vi "Agilent SNA Calibrate.vi"(7 "Agilent SNA & SWP":T6, 8 "error in (no error)":errorcluster, 10 "Parameters to Measure":T2[](array[typedef]) {"Channel" min=1 max=99 step=1; "Parameter"."Stimulus Port" min=1 step=1; "Parameter"."Response Port" min=1 step=1}, 11 "VISA Resource Names":T1) -> (0 "error out":errorcluster {"code" format="%.0x"}, 3 "dup VISA Resource Names":T1)   [LabVIEW 2011]
uses:
  TypeDefs/Agilent SNA VISA.ctl
  TypeDefs/Agilent SNA Instrument Info.ctl
  tests/S Parameter/TypeDefs/SP Parameter to Measure.ctl
  tests/S Parameter/TypeDefs/SP Parameter.ctl
  tests/S Parameter/TypeDefs/SP Calibration State.ctl
  tests/S Parameter/TypeDefs/SP Measurement Format.ctl
  TypeDefs/Agilent SNA Message Mode.ctl
  TypeDefs/Agilent SNA Display Data.ctl
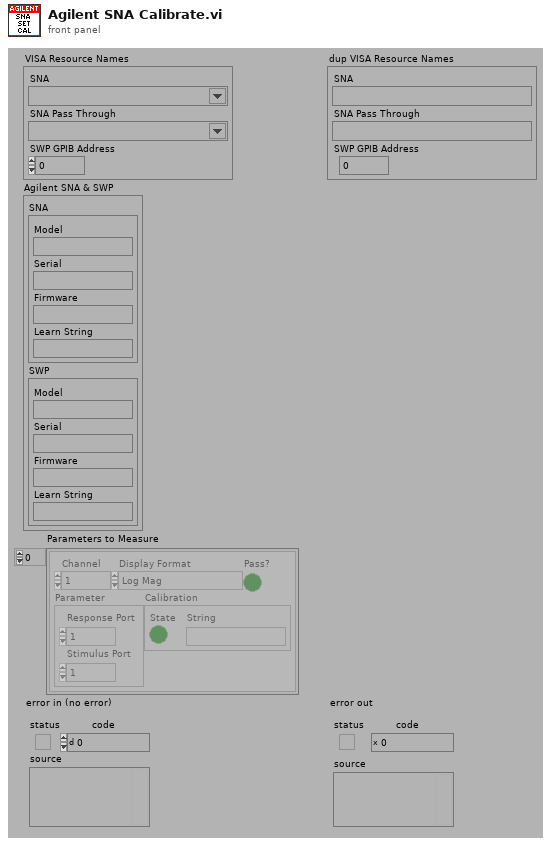
[diagram p1: front panel]
types:
  T1 = typedef "Agilent SNA VISA.ctl" = cluster{"SNA":refnum<visa-resource-name>, "SNA Pass Through":refnum<visa-resource-name>, "SWP GPIB Address":i32}
  T2 = typedef "SP Parameter to Measure.ctl" = cluster{"Channel":i8, "Parameter":T3, "Calibration":T4, "Display Format":T5, "Pass?":bool}
  T3 = typedef "SP Parameter.ctl" = cluster{"Stimulus Port":i8, "Response Port":i8}
  T4 = typedef "SP Calibration State.ctl" = cluster{"State":bool, "String":string}
  T5 = typedef "SP Measurement Format.ctl" = enum32{"Log Mag", "Phase", "Delay", "Smith (R+jX)", "Polar (Re/Im)", "Linear Mag", "SWR", "Real", "Imaginary", "Smith (Lin/Phase)", "Smith (Log/Phase)", "Smith (Real/Imag)", "Smith (G+jB)", "Polar (Lin/Phase)", "Polar (Log/Phase)", "Expanded Phase", "Positive Phase", "Inverted Smith", "Unwrapped Phase", "Power Out", "Power In", "Linear Mag/Phase", "Log Mag/Phase", "Real/Imaginary"}
  T6 = typedef "Agilent SNA Instrument Info.ctl" = cluster{"SNA":cluster{"Model":string, "Serial":string, "Firmware":string, "Learn String":string}, "SWP":cluster{"Model":string, "Serial":string, "Firmware":string, "Learn String":string}}
  T7 = typedef "Agilent SNA Message Mode.ctl" = enum16{"On", "Off"}
  T8 = typedef "Agilent SNA Display Data.ctl" = enum16{"MEAS", "MEM", "MEAS-MEM"}
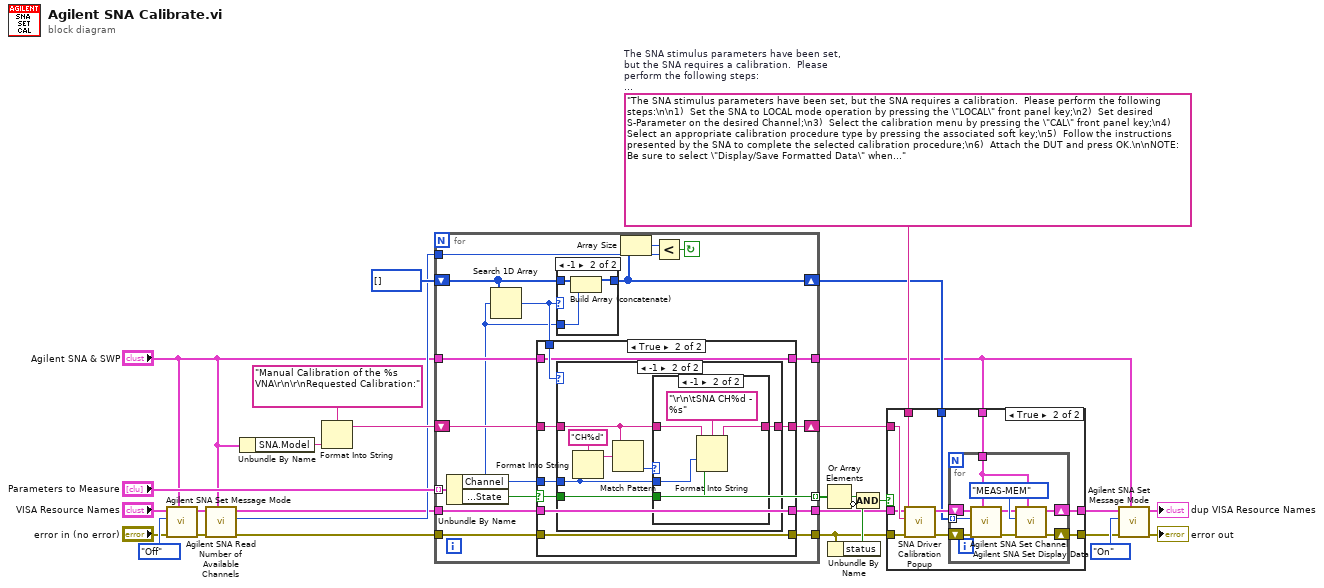
[diagram p0: block diagram]
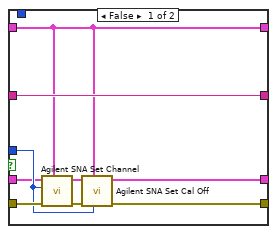
[diagram p3: hidden frame]
diagram:
  w24 = "The SNA stimulus parameters have been set, but the SNA requires a calibration.  Please perform the following steps:\n\n1)  Set the SNA to LOCAL mode operation by pressing the \"LOCAL\" front panel key;\n2)  Set desired S-Parameter on the desired Channel;\n3)  Select the calibration menu by pressing the \"CAL\" front panel key;\n4)  Select an appropriate calibration procedure type by pressing the associated soft key;\n5)  Follow the instructions presented by the SNA to complete the selected calibration procedure;\n6)  Attach the DUT and press OK.\n\nNOTE: Be sure to select \"Display/Save Formatted Data\" when running tests in order to collect the calibrated data."  # The SNA stimulus parameters have been set, but the SNA requires a calibration.  Please perform the following steps:  1)  Set the SNA to LOCAL mode operation by pressing the "LOCAL" front panel key; 2)  Set desired S-Parameter on the desired Channel; 3)  Select the calibration menu by pressing the "CAL" front panel key; 4)  Select an appropriate calibration procedure type by pressing the associated soft key; 5)  Follow the instructions presented by the SNA to complete the selected calibration procedure; 6)  Attach the DUT and press OK.  NOTE: Be sure to select "Display/Save Formatted Data" when running tests in order to collect the calibrated data.
  n1 = call "Agilent SNA Set Message Mode.vi"("Agilent SNA & SWP"="Agilent SNA & SWP", "error in (no error)"="error in (no error)", "Message Mode"=Agilent_SNA_Message_Mode."Off", "VISA Resource Names"="VISA Resource Names") -> ("error out"=w2:errorcluster, "dup VISA Resource Names"=w1:T1)  [unwired: 6 out]
  n2 = call "Agilent SNA Read Number of Available Channels.vi"("Agilent SNA & SWP"="Agilent SNA & SWP", "error in (no error)"=w2, "VISA Resource Names"=w1) -> ("error out"=w22:errorcluster, "Number of Channels"=w21:i8, "dup VISA Resource Names"=w20:T1)  [unwired: 6 out]
  n3 = Unbundle By Name("Agilent SNA & SWP") -> ("SNA.Model"=w27:string)
  n4 = Format Into String(format string="Manual Calibration of the %s VNA\r\n\r\nRequested Calibration:", w27) -> (resulting string=w28:string)  [unwired: 2 in, 1 out]
  n5 = for {
    shift-right: [w45] -> w23
    shift-left: w28 -> [w46]
    tunnel: "Parameters to Measure" -> [w44] mode=indexing
    tunnel: "Agilent SNA & SWP" -> [w42]
    tunnel: w20 -> [w43]
    tunnel: w22 -> [w41]
    tunnel: [w40] -> w15
    shift-right: [w38] -> w13
    shift-left: i8[] [] -> [w39]
    tunnel: w21 -> [w36]
    tunnel: [w34] -> w14
    tunnel: [w32] -> w19 mode=indexing
    tunnel: [w30] -> w5
    stop <- w31 continue-if-true
    n6 = Unbundle By Name(w44) -> ("Channel"=w33:i8, "Calibration.State"=w32:bool)
    n7 = Search 1D Array(1D array=w39, element=w33) -> (index of element=w35:i32)  [unwired: 1 out]
    n8 = case shown="True" w32 {
      selector: w32 -> [_ w64]
      tunnel: w46 -> [w58 w65]
      tunnel: [w58 w67] -> w45
      tunnel: w33 -> [w54 w63]
      tunnel: w43 -> [w53 w61]
      tunnel: w42 -> [w51 w60]
      tunnel: w41 -> [w56 w66]
      tunnel: [w59 w66] -> w40
      tunnel: w35 -> [_ w62]
      tunnel: [w57 w61] -> w34
      tunnel: [w51 w60] -> w30
      frame False {
        n9 = call "Agilent SNA Set Channel.vi"("Agilent SNA & SWP"=w51, "error in (no error)"=w56, "Channel"=w54, "VISA Resource Names"=w53) -> ("error out"=w55:errorcluster, "dup VISA Resource Names"=w52:T1)  [unwired: 6 out]
        n10 = call "Agilent SNA Set Cal Off.vi"("Channel"=w54, "Agilent SNA"=w51, "error in (no error)"=w55, "VISA Resource Names"=w52) -> ("error out"=w59:errorcluster, "dup VISA Resource Names"=w57:T1)  [unwired: 6 out]
      }
      frame True {
        n11 = case shown="-1" w62 {
          tunnel: [w68 w75] -> w67
          tunnel: w65 -> [w68 w74]
          tunnel: w64 -> [_ w73]
          tunnel: w63 -> [_ w71]
          frame Default {
          }
          frame -1 {
            n12 = Format Into String(format string="CH%d", w71) -> (resulting string=w72:string)  [unwired: 2 in, 1 out]
            n13 = Match Pattern(string=w74, regular expression=w72) -> (offset past match=w69:i32)  [unwired: 4 out]
            n14 = case shown="-1" w69 {
              tunnel: [w76 w80] -> w75
              tunnel: w74 -> [w76 w79]
              tunnel: w73 -> [_ w78]
              tunnel: w71 -> [_ w77]
              frame Default {
              }
              frame -1 {
                n15 = Format Into String(format string="\r\n\tSNA CH%d - %s", initial string=w79, w77, w78) -> (resulting string=w80:string)  [unwired: 1 in, 1 out]
              }
            }
          }
        }
      }
    }
    n16 = case shown="-1" w35 {
      tunnel: w39 -> [w47 w50]
      tunnel: [w47 w49] -> w38
      tunnel: w33 -> [_ w48]
      frame Default {
      }
      frame -1 {
        n17 = Build Array (concatenate)(w50, w48) -> (w49:i8[])
      }
    }
    n18 = Array Size(array=w38) -> (size(s)=w37:i32)
    n19 = Less?(x=w37, y=w36) -> (x < y?=w31:bool)
  }
  n20 = Or Array Elements(Boolean array=w19) -> (logical OR=w18:bool)
  n21 = Unbundle By Name(w15) -> ("status"=w17:bool)
  n22 = Compound Arithmetic op=AND(w18, invert w17) -> (w16:bool)
  n23 = case shown="True" w16 {
    tunnel: w24 -> [_ w92]
    tunnel: [w82 w88] -> w3
    tunnel: w23 -> [_ w91]
    tunnel: w15 -> [w82 w90]
    tunnel: w14 -> [w83 w87]
    tunnel: w5 -> [_ w85]
    tunnel: [w83 w86] -> w4
    tunnel: w13 -> [_ w84]
    frame False {
    }
    frame True {
      n24 = call "SNA Driver Calibration Popup.vi"("error in (no error)"=w90, "RequestedCal"=w91, "Message (\"\")"=w92) -> ("error out"=w89:errorcluster)  [unwired: 8 out]
      n25 = for {
        tunnel: w85 -> [w94]
        shift-right: [w101] -> w88
        shift-left: w89 -> [w97]
        shift-right: [w99] -> w86
        shift-left: w87 -> [w98]
        tunnel: w84 -> [w93] mode=indexing
        n26 = call "Agilent SNA Set Channel.vi"("Agilent SNA & SWP"=w94, "error in (no error)"=w97, "Channel"=w93, "VISA Resource Names"=w98) -> ("error out"=w96:errorcluster, "dup VISA Resource Names"=w95:T1)  [unwired: 6 out]
        n27 = call "Agilent SNA Set Display Data.vi"("Agilent SNA & SWP"=w94, "error in (no error)"=w96, "Display Data"=Agilent_SNA_Display_Data."MEAS-MEM", "VISA Resource Names"=w95) -> ("error out"=w101:errorcluster, "dup VISA Resource Names"=w99:T1)  [unwired: 1 in, 5 out]
      }
    }
  }
  n28 = call "Agilent SNA Set Message Mode.vi"("Agilent SNA & SWP"=w5, "error in (no error)"=w3, "Message Mode"=Agilent_SNA_Message_Mode."On", "VISA Resource Names"=w4) -> ("error out"=→"error out":errorcluster, "dup VISA Resource Names"=→"dup VISA Resource Names":T1)  [unwired: 6 out]
